vi "Cntrl Loop Actuator Out 2 MM Comand.vi"(5 "Act Cmds In":dbl[][](array[numeric]), 7 "Number of\nLBCBs In":T1, 11 "error in (no error)":errorcluster) -> (6 "Cmd Out":T2[](array[typedef]), 15 "error out":errorcluster)   [LabVIEW 2013]
uses:
  Act & Cart Commands.ctl
  Data Access Objects/Application/Number Of LBCBs.ctl
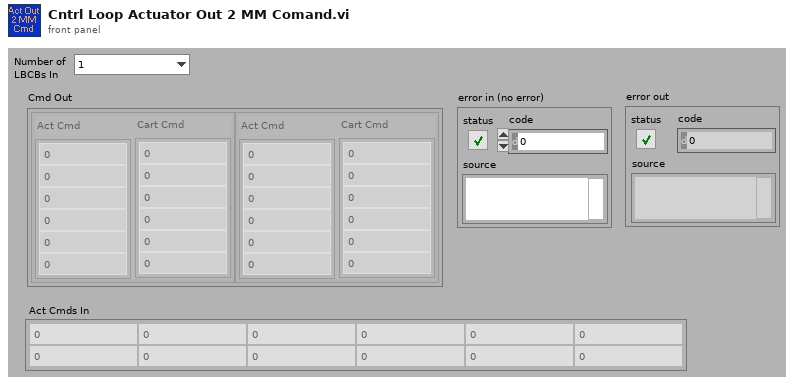
[diagram p1: front panel]
types:
  T1 = typedef "Number Of LBCBs.ctl" = enum16{"1", "2"}
  T2 = typedef "Act & Cart Commands.ctl" = cluster{"Act Cmd":dbl[], "Cart Cmd":dbl[]}
  T3 = enum16{"Cartesian2ActuatorDisplacements", "Actuator2CartesianDisplacements", "Actuators2CartesianForces"}
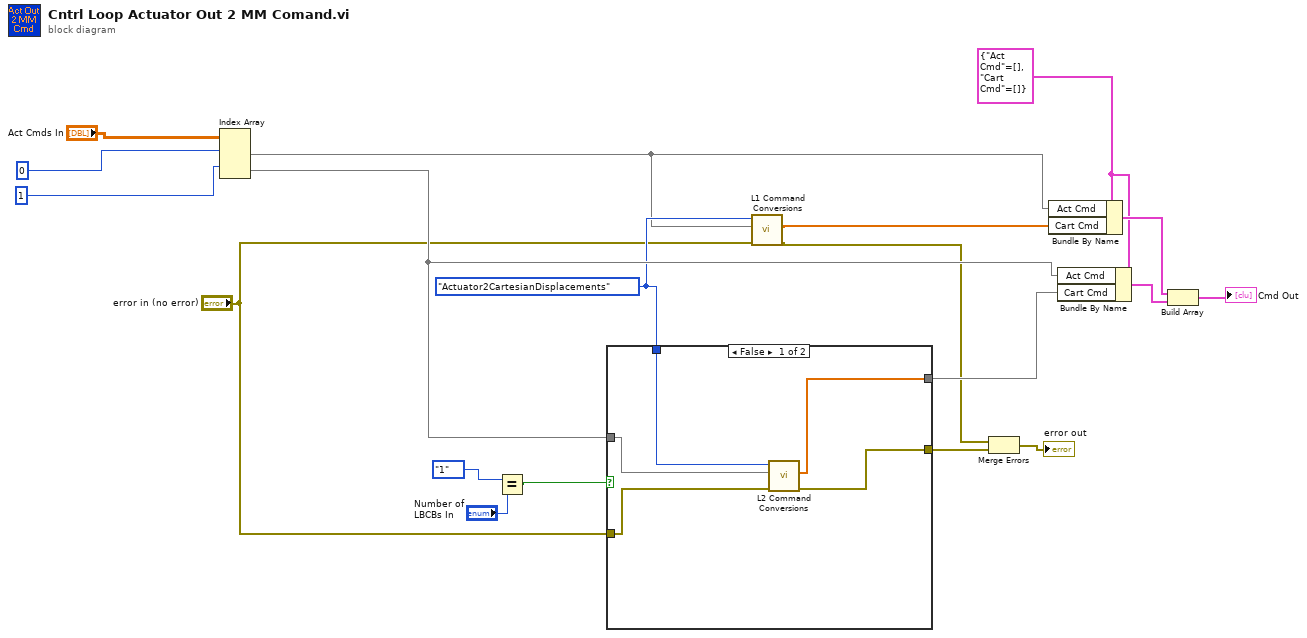
[diagram p0: block diagram]
diagram:
  w5 = T3."Actuator2CartesianDisplacements" ("ConversionOps")
  w10 = T2 {"Act Cmd"=[], "Cart Cmd"=[]} ("L2 Cmd Out")
  n1 = Index Array(array="Act Cmds In", index (row) #1=0 ("index (row)"), index (row) #2=1 ("index (row)")) -> (element #1=w4:dbl[], element #2=w9:dbl[])  [unwired: 2 in]
  n2 = Equal?(x=Number_Of_LBCBs."1", y="Number of\nLBCBs In") -> (x = y?=w15:bool)
  n3 = case shown="False" w15 {
    tunnel: w9 -> [w23 w26]
    tunnel: [w21 w26] -> w8
    tunnel: "error in (no error)" -> [w22 w25]
    tunnel: [w20 w25] -> w7
    tunnel: w5 -> [w24 _]
    frame False {
      n4 = call "L2 Command Conversions.vi"("error in (no error)"=w22, "Inputs"=w23, "ConversionOps"=w24) -> ("error out"=w20:errorcluster, "Outputs"=w21:dbl[])  [unwired: 7 in]
    }
    frame True {
    }
  }
  n5 = call "L1 Command Conversions.vi"("error in (no error)"="error in (no error)", "Inputs"=w4, "ConversionOps"=w5) -> ("error out"=w1:errorcluster, "Outputs"=w2:dbl[])  [unwired: 7 in]
  n6 = Merge Errors(w1, w7) -> (→"error out":errorcluster)
  n7 = Bundle By Name(cluster=w10, "Act Cmd"=w4, "Cart Cmd"=w2) -> (w14:T2)
  n8 = Bundle By Name(cluster=w10, "Act Cmd"=w9, "Cart Cmd"=w8) -> (w18:T2)
  n9 = Build Array(w14, w18) -> (→"Cmd Out":T2[])
